vi "Equi-Ripple BandStop.vi"   [LabVIEW 2010, in "NI_AALBase.lvlib"]
doc: "Generates a bandstop FIR digital filter with equi-ripple characteristics using the Parks-McClellan algorithm and <B>higher pass freq</B>, <B>lower pass freq</B>, <B># of taps</B>, <B>lower stop freq</B>, <B>higher stop freq</B>, and <B>sampling freq: fs</B>. The Equi-Ripple BandStop VI then applies a linear-phase, bandstop filter to the input sequence <B>X</B> using the Convolution VI to obtain <B>Filtered X</B>. Wire data to the <B>X</B> input to determine the polymorphic instance to use or manually select the instance."
uses:
  NI_AALBase.lvlib
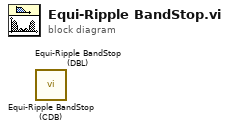
[diagram p0: block diagram]
diagram:
  n1 = call "Equi-Ripple BandStop (CDB).vi"() -> ()  [unwired: 8 in, 2 out]
  n2 = call "Equi-Ripple BandStop (DBL).vi"() -> ()  [unwired: 8 in, 2 out]
